vi "Robot2.vi"() -> ()   [LabVIEW 2016]
uses:
  <vilib>/NXT/Block Support/NXT_InputPort.ctl
  <vilib>/NXT/Subs/LVHSConnector.ctl
  <vilib>/NXT/LegoClasses/BrickReference/BrickReference.lvclass
  <vilib>/NXT/Subs/ColorSensorColors.ctl
panel:
  out "Collor":T1
  in  "Enable State change":bool=TRUE
  in  "Colors and Directions":enum16{"Zero", "Right", "Front", "Left"}[](array[ring])=[enum."Zero", enum."Zero", enum."Zero", enum."Zero", enum."Zero", enum."Zero"]
  in  "Correct":bool
  in  "CS":T2(ring)
  out "NXT/EV3 2":T3
  in  "NXT/EV3":T3
  in  "Sensor - Left":T4=3 items=["Port 1", "Port 2", "Port 3", "Port 4"]
  in  "Sensor - Right":T4=3 items=["Port 1", "Port 2", "Port 3", "Port 4"]
  in  "Gyro Port":T4 items=["Port 1", "Port 2", "Port 3", "Port 4"]
  in  "Motor speed":i32=60
  in  "Kp":i32=1
  in  "Distance to street":dbl
  in  "Color \nSensor Port":T4=2 items=["Port 1", "Port 2", "Port 3", "Port 4"]
  # "black"
  # "blue"
  # "green"
  # "yellow"
  # "red"
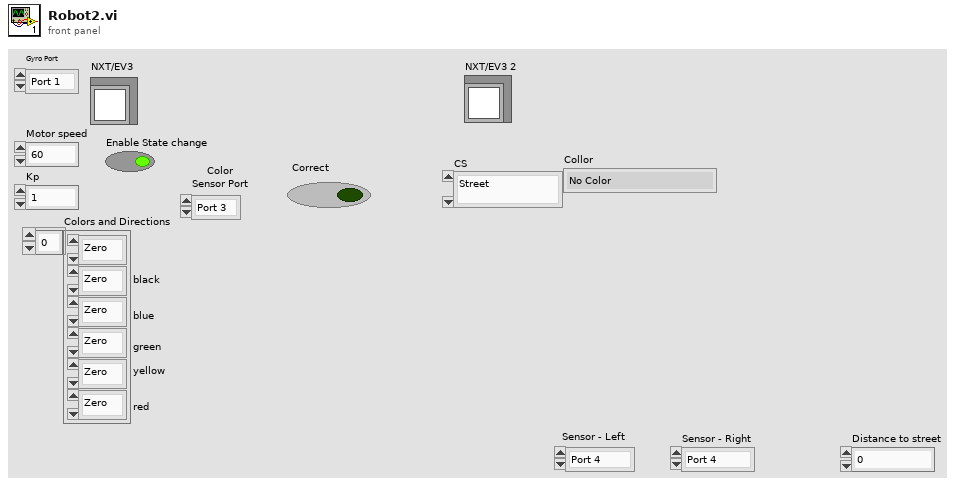
[diagram p1: front panel]
types:
  T1 = typedef "ColorSensorColors.ctl" = enum16{"No Color", "Black", "Blue", "Green", "Yellow", "Red", "White", "Brown"}
  T2 = enum16{"Street", "Intersection", "End", "Stop", "Square", "Delivery"}
  T3 = typedef "LVHSConnector.ctl" = refnum<class "BrickReference.lvclass">
  T4 = typedef "NXT_InputPort.ctl" = u32
  T5 = enum16{"Street", "Intersection", "End", "Stop", "Square"}
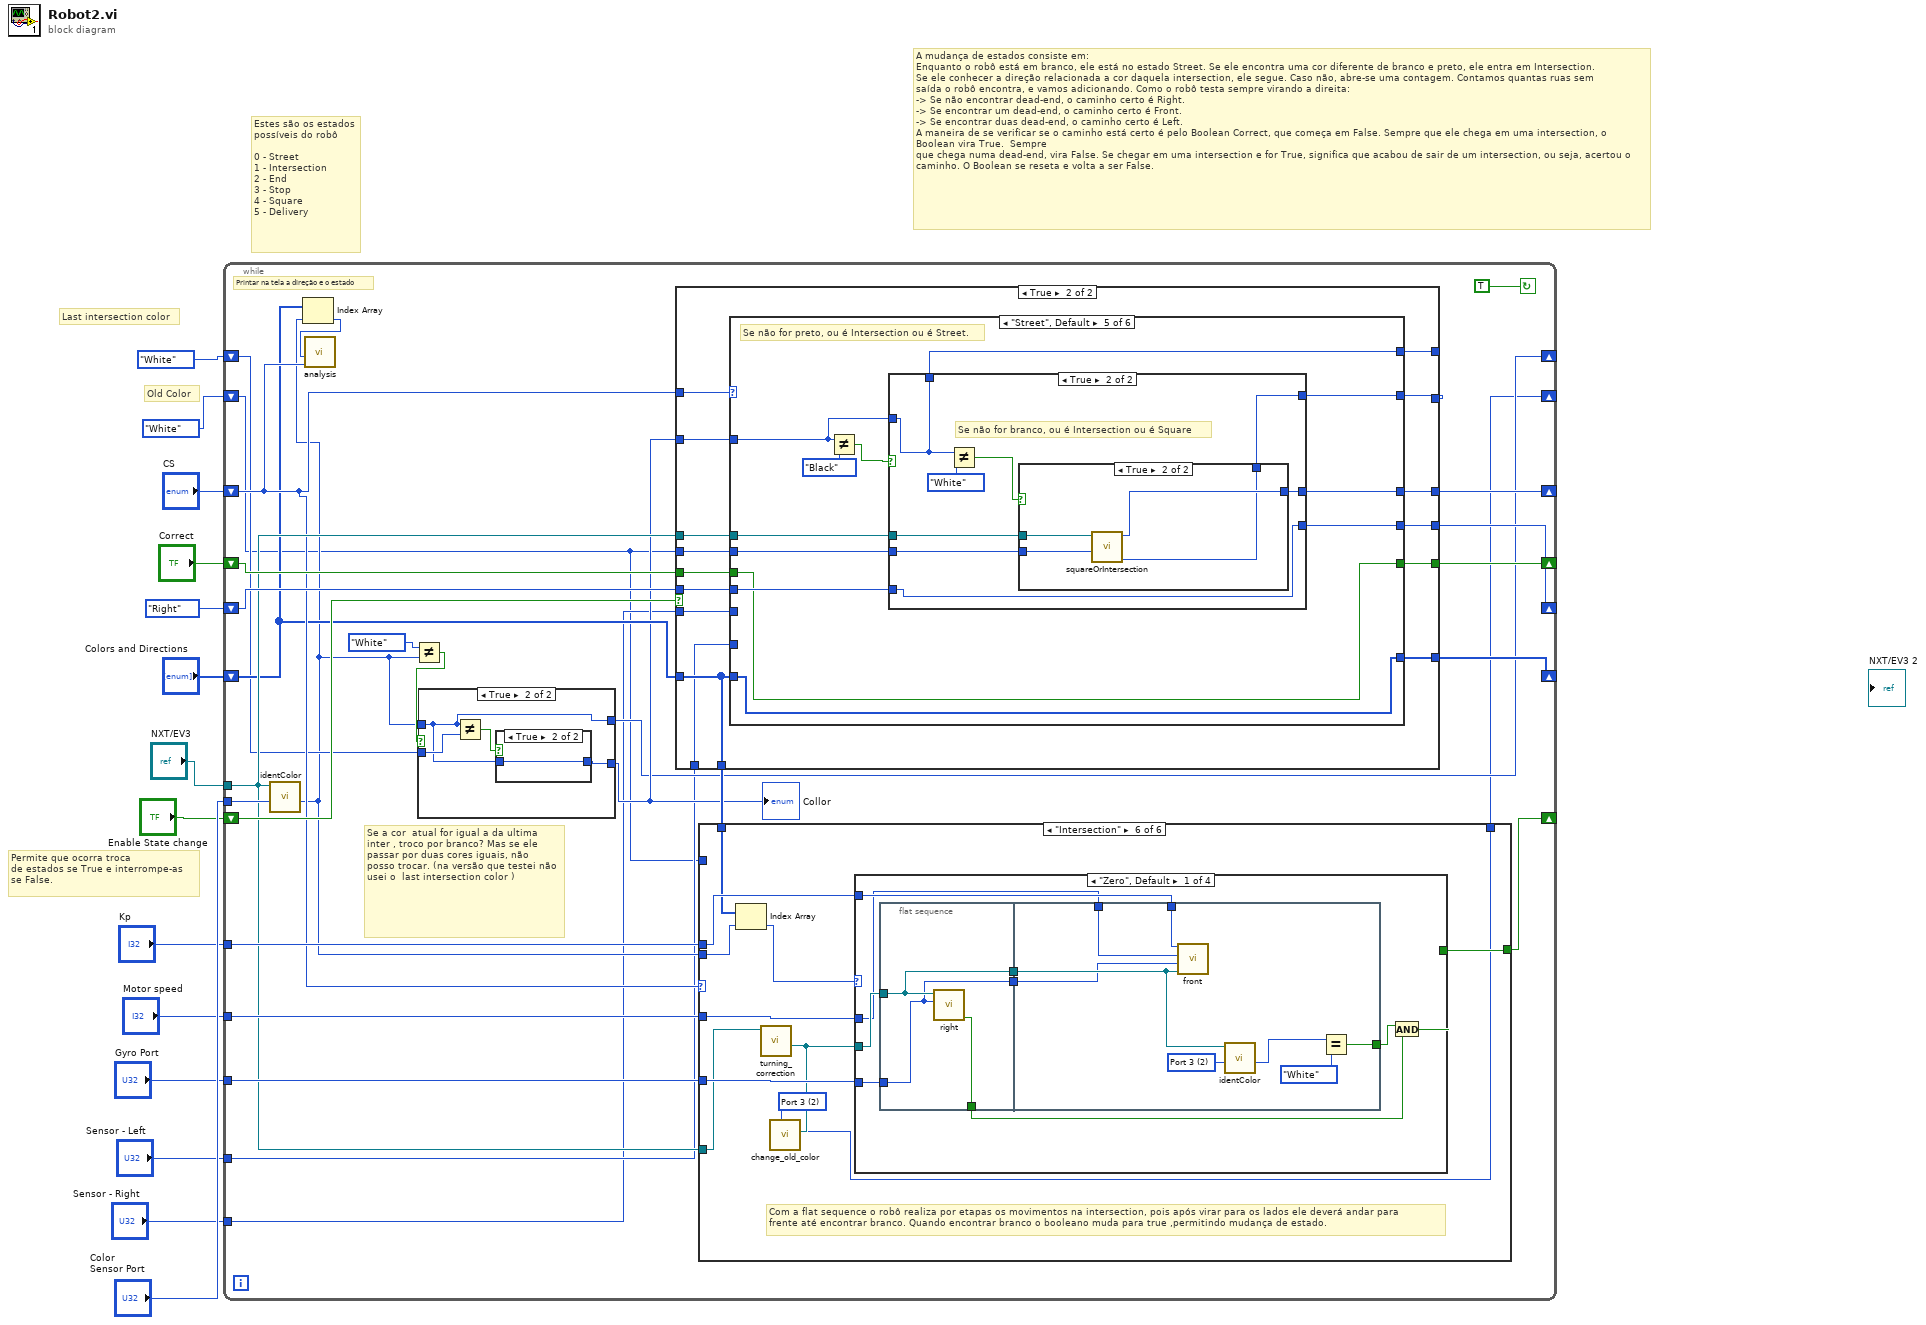
[diagram p0: block diagram]
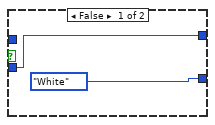
[diagram p2: hidden frame]
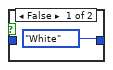
[diagram p3: hidden frame]
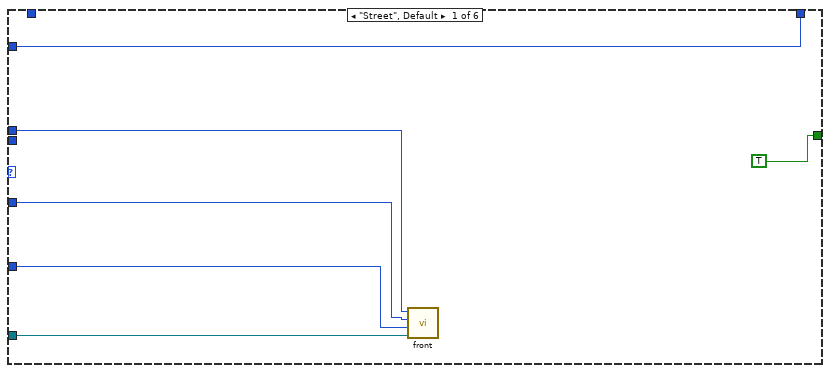
[diagram p4: hidden frame]
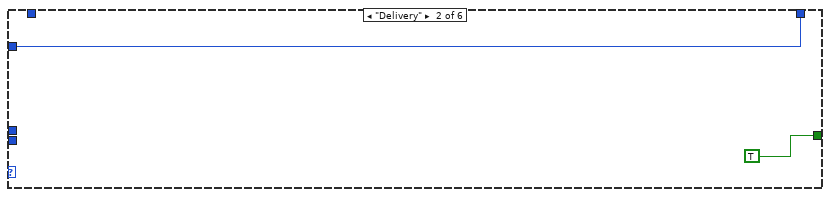
[diagram p5: hidden frame]
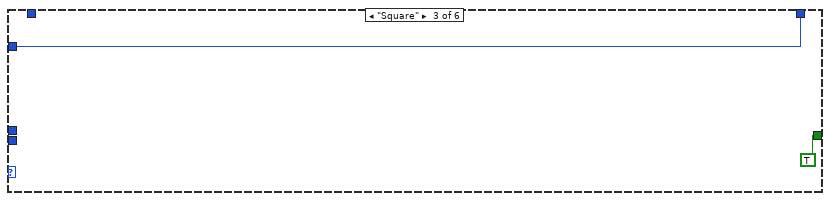
[diagram p6: hidden frame]
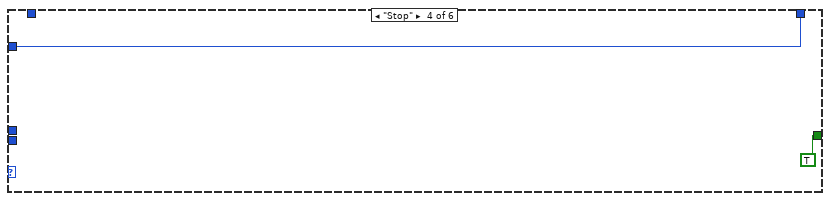
[diagram p7: hidden frame]
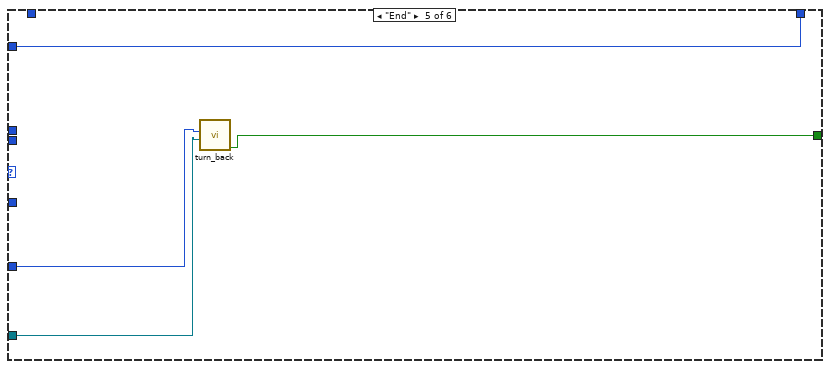
[diagram p8: hidden frame]
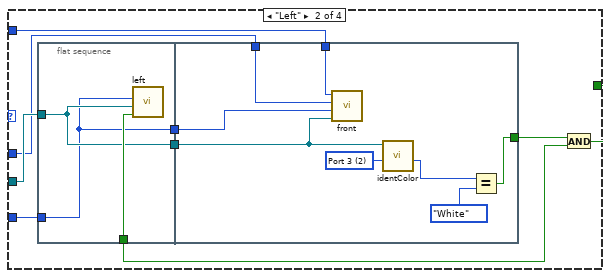
[diagram p9: hidden frame]
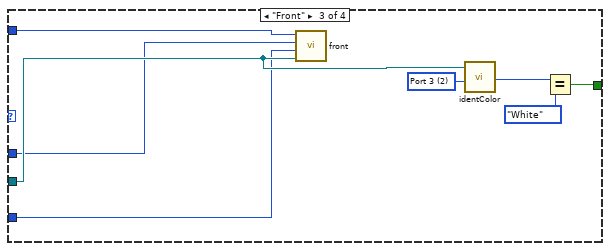
[diagram p10: hidden frame]
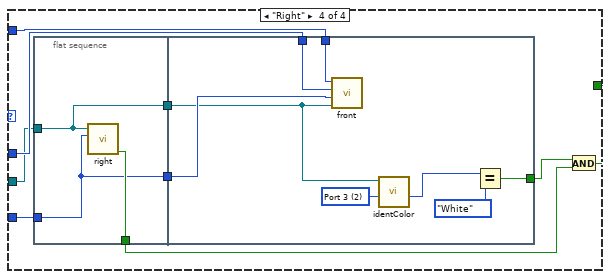
[diagram p11: hidden frame]
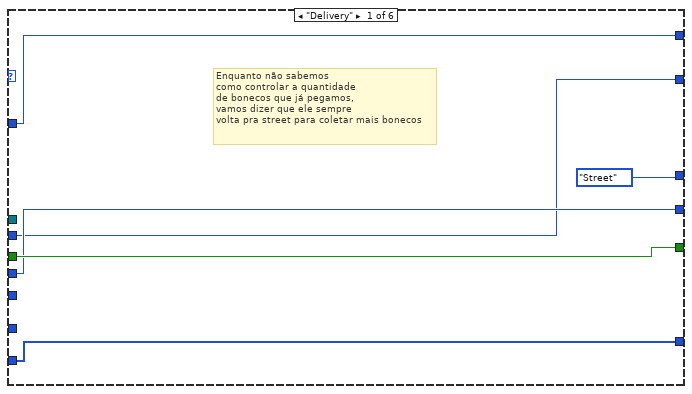
[diagram p13: hidden frame]
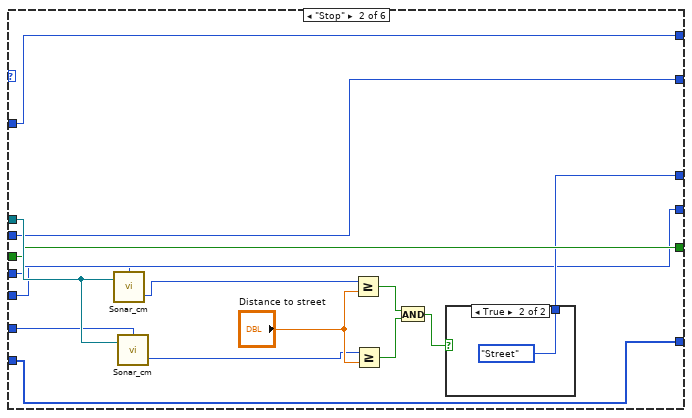
[diagram p14: hidden frame]
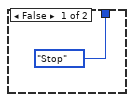
[diagram p15: hidden frame]
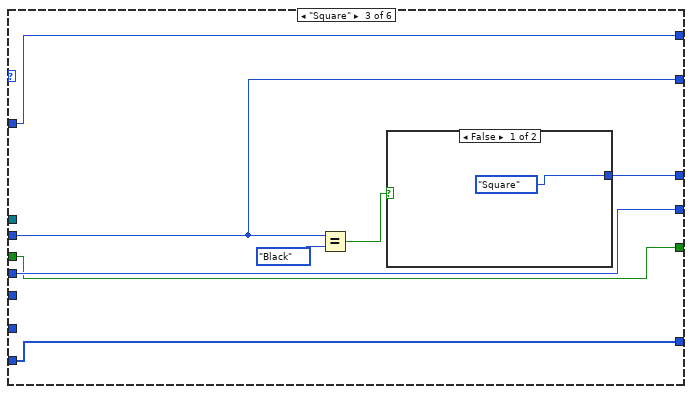
[diagram p16: hidden frame]
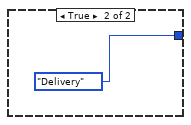
[diagram p17: hidden frame]
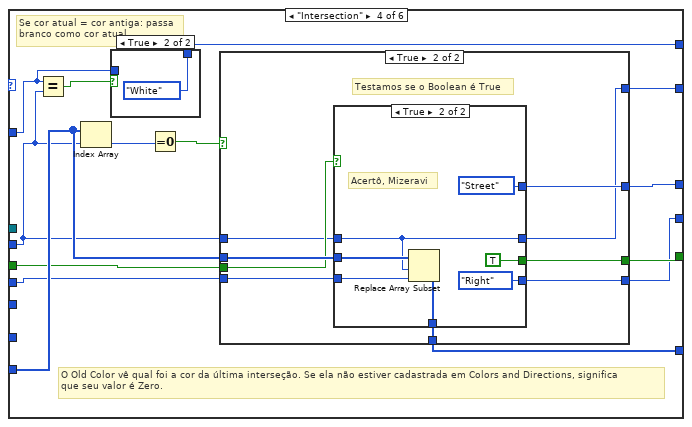
[diagram p18: hidden frame]
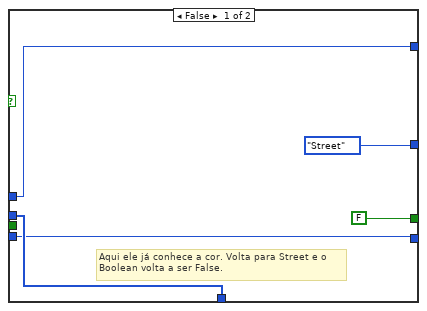
[diagram p20: hidden frame]
diagram:
  # "Last intersection color"
  # "Permite que ocorra troca \nde estados se True e interrompe-as \nse False."
  # "A mudança de estados consiste em:\nEnquanto o robô está em branco, ele está no estado Street. Se ele encontra uma cor diferente de branco e preto, ele entra em Intersection.\nSe ele conhecer a direção relacionada a cor daquela intersection, ele segue. Caso não, abre-se uma contagem. Contamos quantas ruas sem \nsaída o robô encontra, e vamos adicionando. Como o robô testa sempre virando a direita:\n-> Se não encontrar dead-end, o caminho certo é Right.\n-> Se encontrar um dead-end, o caminho certo é Front.\n-> Se encontrar duas dead-end, o caminho certo é Left.\nA maneira de se verificar se o caminho está certo é pelo Boolean Correct, que começa em False. Sempre que ele chega em uma intersection, o Boolean vira True.  Sempre\nque chega numa dead-end, vira False. Se chegar em uma intersection e for True, significa que acabou de sair de um intersection, ou seja, acertou o\ncaminho. O Boolean se reseta e volta a ser False."
  # "Estes são os estados\npossíveis do robô\n\n0 - Street\n1 - Intersection\n2 - End\n3 - Stop\n4 - Square\n5 - Delivery"
  # "Old Color"
  n1 = while {
    tunnel: "NXT/EV3" -> [w31]
    tunnel: "Color \nSensor Port" -> [w42]
    shift-right: [w16] -> _
    shift-left: ColorSensorColors."White" ("Detected Color") -> [w15]
    shift-right: [w41] -> _
    shift-left: "CS" -> [w28]
    shift-right: [w38] -> _
    shift-left: "Correct" -> [w37]
    shift-right: [w39] -> _
    shift-left: enum16{"Zero", "Right", "Front", "Left"}."Right" ("Direction") -> [w40]
    shift-right: [w36] -> _
    shift-left: "Colors and Directions" -> [w24]
    tunnel: "Kp" -> [w34]
    tunnel: "Motor speed" -> [w33]
    tunnel: "Gyro Port" -> [w32]
    shift-right: [w27] -> _
    shift-left: "Enable State change" -> [w35]
    shift-right: [w20] -> _
    shift-left: ColorSensorColors."White" ("Detected Color") -> [w22]
    tunnel: "Sensor - Left" -> [w18]
    tunnel: "Sensor - Right" -> [w17]
    stop <- TRUE continue-if-true
    # "Se a cor  atual for igual a da ultima\ninter , troco por branco? Mas se ele \npassar por duas cores iguais, não \nposso trocar. (na versão que testei não usei o  last intersection color )"
    # "Printar na tela a direção e o estado"
    n2 = call "identColor.vi"("Port (Port 1)"=w42, "NXT/EV3"=w31) -> ("Collor"=w19:T1)  [unwired: 9 in]
    n3 = Index Array(array=w24, index=w19) -> (element=w23:enum16{"Zero", "Right", "Front", "Left"})
    n4 = call "analysis.vi"("CS 2"=w28, "Direction"=w23) -> ()  [unwired: 10 in]
    n5 = Not Equal?(x=ColorSensorColors."White" ("Detected Color"), y=w19) -> (x != y?=w25:bool)
    n6 = case shown="True" w25 {
      tunnel: [ColorSensorColors."White" ("Detected Color") w47] -> w21
      tunnel: w19 -> [_ w45]
      tunnel: w22 -> [w43 w46]
      tunnel: [w43 w45] -> w20
      frame False {
      }
      frame True {
        n7 = Not Equal?(x=w45, y=w46) -> (x != y?=w48:bool)
        n8 = case shown="True" w48 {
          tunnel: [ColorSensorColors."White" ("Detected Color") w50] -> w47
          tunnel: w45 -> [_ w50]
          frame False {
          }
          frame True {
          }
        }
      }
    }
    "Collor" <- w21
    n9 = case shown="True" w35 {
      tunnel: w21 -> [w150 w166]
      tunnel: w31 -> [_ w165]
      tunnel: [w149 w164] -> w41
      tunnel: w15 -> [w146 w163]
      tunnel: w40 -> [w148 w162]
      tunnel: [w148 w161] -> w39
      tunnel: [w147 w160] -> w38
      tunnel: w24 -> [w151 w155]
      tunnel: w37 -> [w147 w159]
      tunnel: [w151 w158] -> w36
      tunnel: [w150 w157] -> _
      tunnel: w28 -> [w149 w156]
      tunnel: [w151 w155] -> w30
      tunnel: [w146 w154] -> _
      tunnel: w18 -> [_ w153]
      tunnel: w17 -> [_ w152]
      frame False {
      }
      frame True {
        n10 = case shown="\"Street\", Default" w156 {
          tunnel: w166 -> [w171 w179 w194 w201 w251 w277]
          tunnel: w165 -> [_ w181 _ _ w250 _]
          tunnel: [enum16{"Street", "Intersection", "End", "Stop"}."Street" ("CS") w178 w195 w206 w249 enum16{"Street", "Intersection", "End"}."Street" ("CS")] -> w164
          tunnel: w163 -> [w167 w175 w190 w204 w248 w276]
          tunnel: w162 -> [w169 w177 w192 w209 w247 w278]
          tunnel: [w169 w177 w192 w207 w246 w278] -> w161
          tunnel: [w170 w180 w191 w208 w244 FALSE] -> w160
          tunnel: w155 -> [w168 w176 w193 w211 w245 w279]
          tunnel: w159 -> [w170 w180 w191 w210 w244 _]
          tunnel: [w168 w176 w193 w205 w245 w279] -> w158
          tunnel: [w171 w179 w194 w202 w243 w277] -> w157
          tunnel: [w167 w175 w190 w200 w242 w276] -> w154
          tunnel: w153 -> [_ w174 _ _ _ _]
          tunnel: w152 -> [_ w173 _ _ _ _]
          frame "Delivery" {
            # "Enquanto não sabemos\ncomo controlar a quantidade\nde bonecos que já pegamos,\nvamos dizer que ele sempre\nvolta pra street para coletar mais bonecos"
          }
          frame "Stop" {
            n11 = call <vilib>:"Sonar_cm.vi"("NXT/EV3"=w181, "Port (Port 4)"=w173) -> ("Distance (cm)"=w183:i16)  [unwired: 1 in, 1 out]
            n12 = call <vilib>:"Sonar_cm.vi"("NXT/EV3"=w181, "Port (Port 4)"=w174) -> ("Distance (cm)"=w182:i16)  [unwired: 1 in, 1 out]
            n13 = Greater Or Equal?(x=w183, y="Distance to street") -> (x >= y?=w185:bool)
            n14 = Greater Or Equal?(x=w182, y="Distance to street") -> (x >= y?=w186:bool)
            n15 = And(x=w185, y=w186) -> (x .and. y?=w184:bool)
            n16 = case shown="True" w184 {
              tunnel: [enum16{"Street", "Intersection", "End", "Stop"}."Stop" ("CS") enum16{"Street", "Intersection", "End", "Stop"}."Street" ("CS")] -> w178
              frame False {
              }
              frame True {
              }
            }
          }
          frame "Square" {
            n17 = Equal?(x=w190, y=ColorSensorColors."Black") -> (x = y?=w196:bool)
            n18 = case shown="False" w196 {
              tunnel: [T2."Square" ("CS") T2."Delivery" ("CS")] -> w195
              frame False {
              }
              frame True {
              }
            }
          }
          frame "Intersection" {
            # "Se cor atual = cor antiga: passa\nbranco como cor atual."
            # "O Old Color vê qual foi a cor da última interseção. Se ela não estiver cadastrada em Colors and Directions, significa\nque seu valor é Zero."
            n19 = Equal?(x=w201, y=w204) -> (x = y?=w203:bool)
            n20 = Index Array(array=w211, index=w204) -> (element=w212:enum16{"Zero", "Right", "Front", "Left"})
            n21 = case shown="True" w203 {
              tunnel: [w214 ColorSensorColors."White" ("Detected Color")] -> w202
              tunnel: w201 -> [w214 _]
              frame False {
              }
              frame True {
              }
            }
            n22 = Equal To 0?(x=w212) -> (x = 0?=w213:bool)
            n23 = case shown="True" w213 {
              tunnel: w211 -> [w218 w229]
              tunnel: w210 -> [_ w228]
              tunnel: w204 -> [w216 w227]
              tunnel: w209 -> [w217 w226]
              tunnel: [FALSE w225] -> w208
              tunnel: [w217 w224] -> w207
              tunnel: [enum16{"Street", "Intersection", "End"}."Street" ("CS") w223] -> w206
              tunnel: [w218 w222] -> w205
              tunnel: [w216 w221] -> w200
              frame False {
                # "Aqui ele já conhece a cor. Volta para Street e o \nBoolean volta a ser False."
              }
              frame True {
                # "Testamos se o Boolean é True"
                n24 = case shown="True" w228 {
                  tunnel: w229 -> [w232 w241]
                  tunnel: w227 -> [w230 w235]
                  tunnel: w226 -> [w231 w240]
                  tunnel: [TRUE TRUE] -> w225
                  tunnel: [w231 enum16{"Zero", "Right", "Front", "Left"}."Right" ("Direction")] -> w224
                  tunnel: [enum16{"Street", "Intersection", "End"}."Street" ("CS") enum16{"Street", "Intersection", "End"}."Street" ("CS")] -> w223
                  tunnel: [w232 w236] -> w222
                  tunnel: [w230 w235] -> w221
                  frame False {
                    # "Volta para Street e o Boolean\nvira True; o robô ainda não\nacertou."
                  }
                  frame True {
                    # "Acertô, Mizeravi"
                    n25 = Replace Array Subset(array=w241, new element=w240, index=w235) -> (w236:enum16{"Zero", "Right", "Front", "Left"}[])
                  }
                }
              }
            }
          }
          frame "Street", Default {
            # "Se não for preto, ou é Intersection ou é Street."
            n26 = Not Equal?(x=w251, y=ColorSensorColors."Black" ("Detected Color")) -> (x != y?=w252:bool)
            n27 = case shown="True" w252 {
              tunnel: w251 -> [w255 w260]
              tunnel: w250 -> [_ w264]
              tunnel: [enum16{"Street", "Intersection", "End"}."End" ("CS") w263] -> w249
              tunnel: w248 -> [w254 w262]
              tunnel: w247 -> [w257 w261]
              tunnel: [w256 w261] -> w246
              tunnel: [w255 w260] -> w243
              tunnel: [w254 w259] -> w242
              frame False {
                # "Nesse caso, ele chegou numa dead-end; vai para o estado End\ne adiciona um no contador."
                n28 = Increment(x=w257) -> (x+1=w256:enum16{"Zero", "Right", "Front", "Left"})
              }
              frame True {
                # "Se não for branco, ou é Intersection ou é Square"
                n29 = Not Equal?(x=w260, y=ColorSensorColors."White" ("Detected Color")) -> (x != y?=w265:bool)
                n30 = case shown="True" w265 {
                  tunnel: w264 -> [w268 w275]
                  tunnel: [w271 w274] -> w263
                  tunnel: w262 -> [w267 w273]
                  tunnel: [w267 w272] -> w259
                  frame False {
                    # "Ou ele vai para Stop ou continua em Street"
                    n31 = call <vilib>:"Sonar_cm.vi"("NXT/EV3"=w268) -> ("Distance (cm)"=w269:i16)  [unwired: 2 in, 1 out]
                    n32 = call <vilib>:"Sonar_cm.vi"("NXT/EV3"=w268) -> ("Distance (cm)"=w270:i16)  [unwired: 2 in, 1 out]
                    n33 = call "toStop.vi"("Left"=w269, "Right"=w270) -> ("Next State"=w271:enum16{"Street", "Intersection", "End", "Stop"})  [unwired: 13 in]
                  }
                  frame True {
                    n34 = call "squareOrIntersection.vi"("Old Color IN"=w273, "NXT/EV3"=w275) -> ("Old Color OUT"=w272:T1, "CS"=w274:T5)  [unwired: 8 in]
                  }
                }
              }
            }
          }
          frame "End" {
            # "Depois de um End, ele sempre volta para Street, e o Boolean vira False"
          }
        }
      }
    }
    n35 = case shown="\"Intersection\"" w28 {
      tunnel: [TRUE TRUE ("x = y?") TRUE ("x = y?") TRUE ("x = y?") w66 w72] -> w27
      tunnel: w34 -> [w55 _ _ _ _ w76]
      tunnel: w33 -> [w54 _ _ _ _ w75]
      tunnel: w32 -> [w53 _ _ _ w64 w77]
      tunnel: w31 -> [w52 _ _ _ w65 w71]
      tunnel: w30 -> [_ _ _ _ _ w74]
      tunnel: w19 -> [_ _ _ _ _ w70]
      tunnel: [w51 w57 w59 w61 w63 w67] -> w16
      tunnel: w15 -> [w51 w57 w59 w61 w63 _]
      frame "Street", Default {
        n36 = call "front.vi"("NXT/EV3"=w52, "Gyro Port"=w53, "Motor speed"=w54, "Kp"=w55) -> ()  [unwired: 8 in]
      }
      frame "Delivery" {
      }
      frame "Square" {
      }
      frame "Stop" {
      }
      frame "End" {
        n37 = call "turn_back.vi"("NXT/EV3"=w65, "Gyro Port"=w64) -> ("x = y?"=w66:bool)  [unwired: 9 in]
      }
      frame "Intersection" {
        w69 = T4 2 items=["Port 1", "Port 2", "Port 3", "Port 4"] ("Port (Port 3)")
        # "Com a flat sequence o robô realiza por etapas os movimentos na intersection, pois após virar para os lados ele deverá andar para\nfrente até encontrar branco. Quando encontrar branco o booleano muda para true ,permitindo mudança de estado."
        n38 = Index Array(array=w74, index=w70) -> (element=w73:enum16{"Zero", "Right", "Front", "Left"})
        n39 = call "turning_correction.vi"("NXT/EV3"=w71) -> ("NXT/EV3 2"=w68:T3)  [unwired: 10 in]
        n40 = call "change_old_color.vi"("Port (Port 3)"=w69, "NXT/EV3"=w68) -> ("Detected Color"=w67:T1)  [unwired: 9 in]
        n41 = case shown="\"Zero\", Default" w73 {
          tunnel: [w85 w105 w123 w126] -> w72
          tunnel: w68 -> [w84 w104 w122 w129]
          tunnel: w77 -> [w83 w101 w118 w130]
          tunnel: w76 -> [w80 w100 w120 w132]
          tunnel: w75 -> [w79 w99 w119 w131]
          frame "Zero", Default {
            n42 = flat-sequence {
              tunnel: w84 -> [w88]
              tunnel: w83 -> [w87]
              tunnel: [w89] -> w82
              tunnel: [w88] -> w81
              tunnel: [w87] -> w78
              tunnel: [w96] -> w86
              tunnel: w81 -> [w94]
              tunnel: w80 -> [w93]
              tunnel: w79 -> [w92]
              tunnel: w78 -> [w91]
              frame #0 {
                n43 = call "right.vi"("Gyro Port"=w87, "NXT/EV3"=w88) -> ("x = y?"=w89:bool)  [unwired: 9 in]
              }
              frame #1 {
                w90 = T4 2 items=["Port 1", "Port 2", "Port 3", "Port 4"] ("Port (Port 1)")
                n44 = call "front.vi"("NXT/EV3"=w94, "Gyro Port"=w91, "Motor speed"=w92, "Kp"=w93) -> ()  [unwired: 8 in]
                n45 = call "identColor.vi"("Port (Port 1)"=w90, "NXT/EV3"=w94) -> ("Collor"=w95:T1)  [unwired: 9 in]
                n46 = Equal?(x=w95, y=ColorSensorColors."White") -> (x = y?=w96:bool)
              }
            }
            n47 = And(x=w86, y=w82) -> (x .and. y?=w85:bool)
          }
          frame "Left" {
            n48 = flat-sequence {
              tunnel: [w109] -> w106
              tunnel: w104 -> [w108]
              tunnel: [w108] -> w102
              tunnel: w101 -> [w107]
              tunnel: [w107] -> w98
              tunnel: [w115] -> w103
              tunnel: w102 -> [w114]
              tunnel: w100 -> [w113]
              tunnel: w99 -> [w112]
              tunnel: w98 -> [w111]
              frame #0 {
                n49 = call "left.vi"("NXT/EV3"=w108, "Gyro Port"=w107) -> ("x = y?"=w109:bool)  [unwired: 9 in]
              }
              frame #1 {
                w110 = T4 2 items=["Port 1", "Port 2", "Port 3", "Port 4"] ("Port (Port 1)")
                n50 = call "front.vi"("NXT/EV3"=w114, "Gyro Port"=w111, "Motor speed"=w112, "Kp"=w113) -> ()  [unwired: 8 in]
                n51 = call "identColor.vi"("Port (Port 1)"=w110, "NXT/EV3"=w114) -> ("Collor"=w116:T1)  [unwired: 9 in]
                n52 = Equal?(x=w116, y=ColorSensorColors."White") -> (x = y?=w115:bool)
              }
            }
            n53 = And(x=w103, y=w106) -> (x .and. y?=w105:bool)
          }
          frame "Front" {
            w121 = T4 2 items=["Port 1", "Port 2", "Port 3", "Port 4"] ("Port (Port 1)")
            n54 = call "front.vi"("NXT/EV3"=w122, "Gyro Port"=w118, "Motor speed"=w119, "Kp"=w120) -> ()  [unwired: 8 in]
            n55 = call "identColor.vi"("Port (Port 1)"=w121, "NXT/EV3"=w122) -> ("Collor"=w124:T1)  [unwired: 9 in]
            n56 = Equal?(x=w124, y=ColorSensorColors."White") -> (x = y?=w123:bool)
          }
          frame "Right" {
            n57 = flat-sequence {
              tunnel: [w137] -> w133
              tunnel: w130 -> [w136]
              tunnel: w129 -> [w135]
              tunnel: [w136] -> w128
              tunnel: [w135] -> w127
              tunnel: [w144] -> w134
              tunnel: w132 -> [w141]
              tunnel: w131 -> [w140]
              tunnel: w128 -> [w139]
              tunnel: w127 -> [w138]
              frame #0 {
                n58 = call "right.vi"("Gyro Port"=w136, "NXT/EV3"=w135) -> ("x = y?"=w137:bool)  [unwired: 9 in]
              }
              frame #1 {
                w142 = T4 2 items=["Port 1", "Port 2", "Port 3", "Port 4"] ("Port (Port 1)")
                n59 = call "front.vi"("NXT/EV3"=w138, "Gyro Port"=w139, "Motor speed"=w140, "Kp"=w141) -> ()  [unwired: 8 in]
                n60 = call "identColor.vi"("Port (Port 1)"=w142, "NXT/EV3"=w138) -> ("Collor"=w143:T1)  [unwired: 9 in]
                n61 = Equal?(x=w143, y=ColorSensorColors."White") -> (x = y?=w144:bool)
              }
            }
            n62 = And(x=w134, y=w133) -> (x .and. y?=w126:bool)
          }
        }
      }
    }
  }
